vi "Wait On Occurrence_.vi"(8 "error in":errorcluster, 9 "ms timeout (-1)":i32=-1, 10 "Occurrence User Event":refnum<user-event>, 11 "Occurrence":refnum<event-registration>) -> (0 "error out":errorcluster)   [LabVIEW 2019, in "grpc-lvsupport.lvlib"]
uses:
  grpc-lvsupport.lvlib
  Server API/Server/Get Server Debug DLL Path.vi
  <vilib>/Utility/error.llb/Error Cluster From Error Code.vi
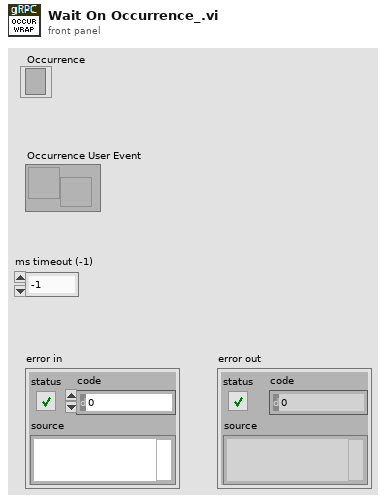
[diagram p1: front panel]
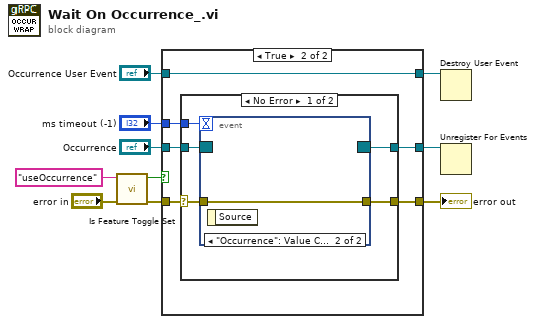
[diagram p0: block diagram]
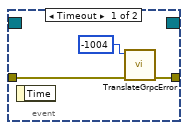
[diagram p3: hidden frame]
diagram:
  n1 = call "Is Feature Toggle Set.vi"("error in (no error)"="error in", "Feature Toggle"="useOccurrence" ("key")) -> ("error out"=w6:errorcluster, "Is Set"=w7:bool)  [unwired: 8 in]
  n2 = case shown="True" w7 {
    tunnel: "Occurrence" -> [w12 w19]
    tunnel: "ms timeout (-1)" -> [_ w18]
    tunnel: [w13 w17] -> w4
    tunnel: w6 -> [w13 w16]
    tunnel: [w12 w15] -> w3
    tunnel: [w11 w14] -> w1
    tunnel: "Occurrence User Event" -> [w11 w14]
    frame False {
    }
    frame True {
      n3 = case shown="No Error" w16 {
        selector: w16 -> [w24 w30]
        tunnel: [w23 w30] -> w17
        tunnel: w19 -> [w21 w29]
        tunnel: w18 -> [w22 _]
        tunnel: [w20 w29] -> w15
        frame No Error {
          n4 = event shown="[1] \"Occurrence\": Value Change" {
            selector: w21 -> [_ _]
            dyn-events: [_ _] -> w20
            timeout: w22 -> [_ _]
            tunnel: w24 -> [w27 w28]
            tunnel: [w26 w28] -> w23
            event Timeout {
              n5 = event-data() -> ()  [unwired: 1 in, 1 out]
              n6 = call "TranslateGrpcError.vi"("error in"=w27, "Error Code"=-1004) -> ("error out"=w26:errorcluster)  [unwired: 9 in]
            }
            event "Occurrence": Value Change {
              n7 = event-data() -> ()  [unwired: 1 in, 1 out]
            }
          }
        }
        frame Error {
        }
      }
    }
  }
  "error out" <- w4
  n8 = Destroy User Event(user event=w1) -> ()  [unwired: 1 in, 1 out]
  n9 = Unregister For Events(event registration refnum=w3) -> ()  [unwired: 1 in, 1 out]
